vi "SP_Production_Count_MonthWise.vi"(8 "error in (no error)":errorcluster) -> (0 "error out":errorcluster)   [LabVIEW 2017]
uses:
  <vilib>/Math Plots/3D Math Plots/3D Pie/3D Pie XCtrl/3D Pie.xctl
  <vilib>/addons/database/Connection.llb/DB Tools Open Connec (Path).vi
  <vilib>/addons/database/Connection.llb/Conn Execute.vi
  <vilib>/addons/database/Recordset.llb/Rec Fetch Recordset Data (R).vi
  <vilib>/addons/database/Recordset.llb/Rec Destroy - Connection.vi
  <vilib>/Math Plots/3D Math Plots/3D Pie/3D Pie Datatype/Public/Plot Helper (Vector).vi
  <vilib>/addons/database/NI_Database_API.lvlib
  <vilib>/Math Plots/3D Math Plots/3D Pie/3D Pie Datatype/3D Pie Datatype.lvclass
panel:
  out "Station size":i32
  in  "Tab Control":enum32{"Data", "Graph"}(tab)
  out "Table":string[][](table)
  out "3D Pie":refnum<class "3D Plot Datatype.lvclass">[](xcontrol)
  out "All Days":string[](array[string])
  in  "Select Year":string(combo)
  in  "Select Month":string(combo)
  out "Station Count":i32
  out "All Shifts":bool
  in  "Cancel Button - Archive":bool
  in  "Download 2":bool
  in  "Get Rport 2":bool
  in  "Shift":string(combo)
  in  "Station":string(combo)
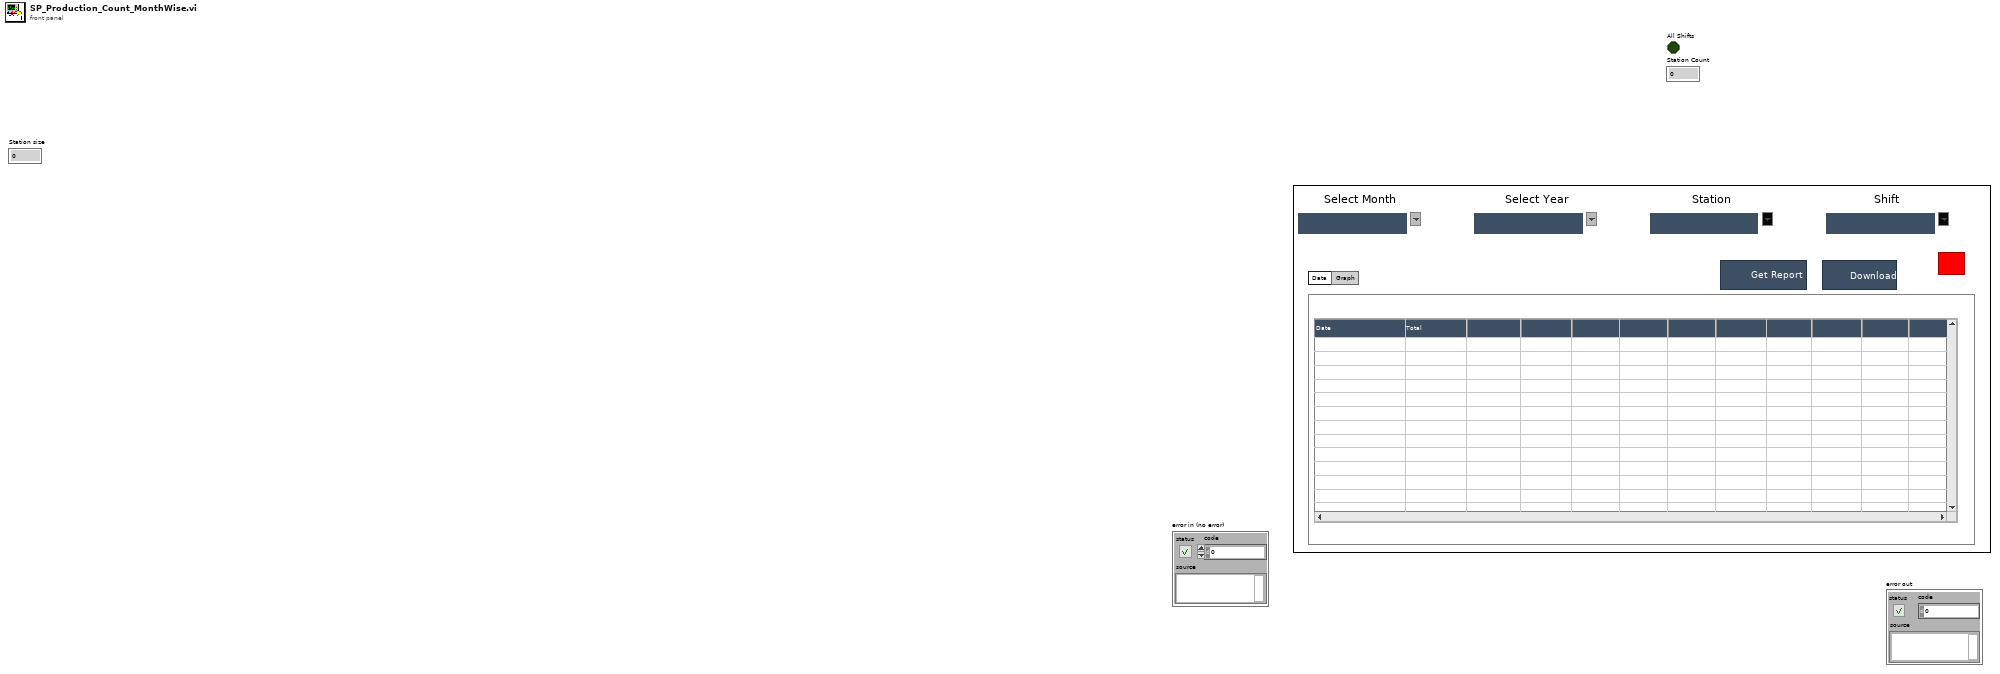
[diagram p1: front panel]
types:
  T1 = typedef "NI_Database_API.lvlib/Conn ObjectReference.ctl" = refnum<k1>
  T2 = typedef "NI_Database_API.lvlib/Rec ObjectReference.ctl" = refnum<k1>
  T3 = enum32{"invalid app kind", "Development System", "Run Time System", "Student Edition", "Embedded LabVIEW", "Evaluation", "Custom"}
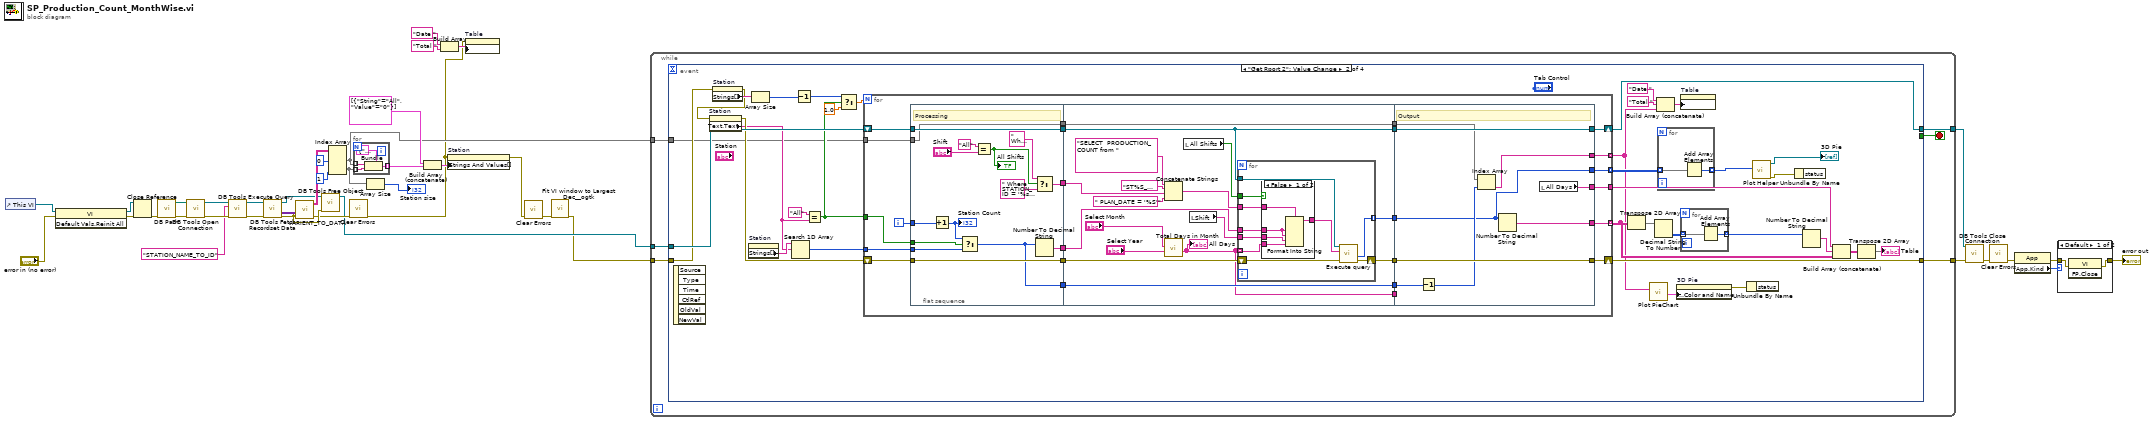
[diagram p0: block diagram]
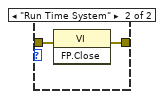
[diagram p2: hidden frame]
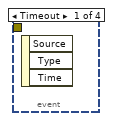
[diagram p3: hidden frame]
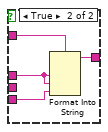
[diagram p4: hidden frame]
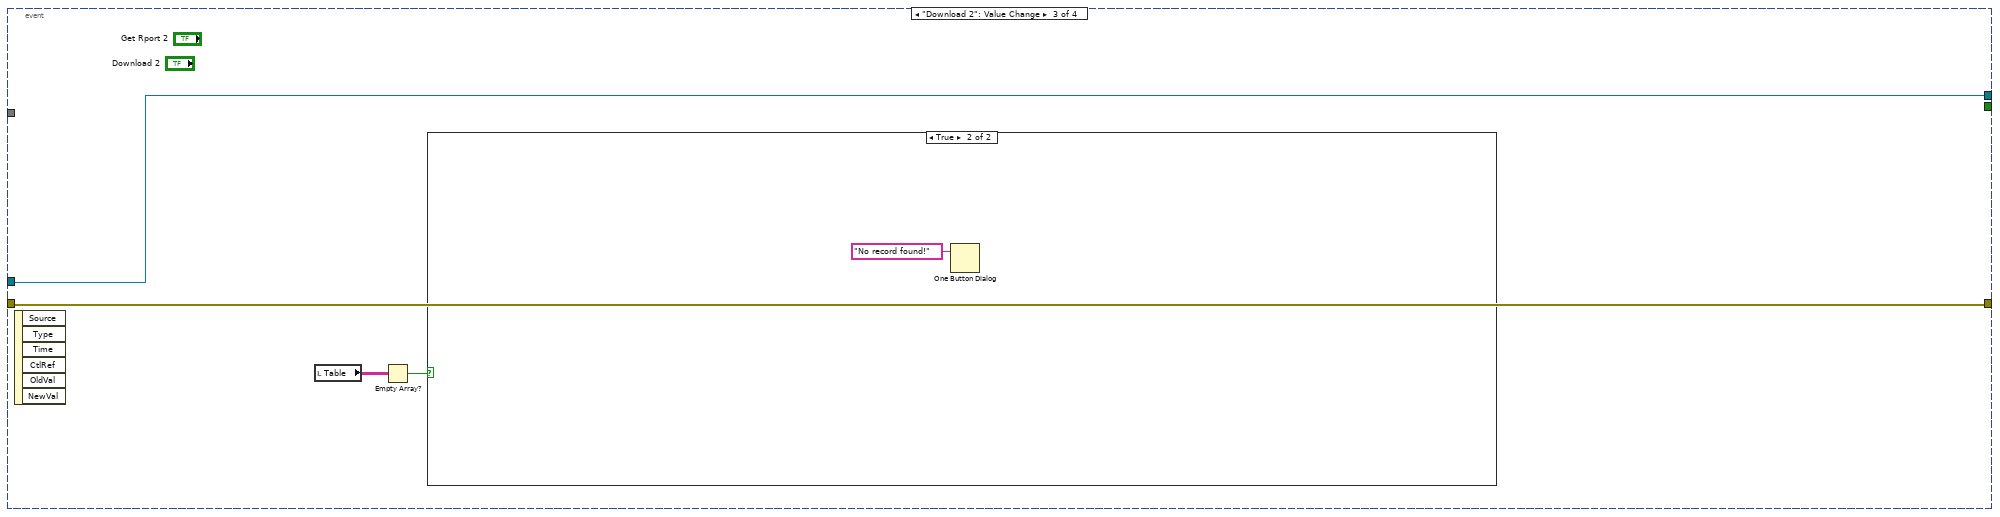
[diagram p5: hidden frame]
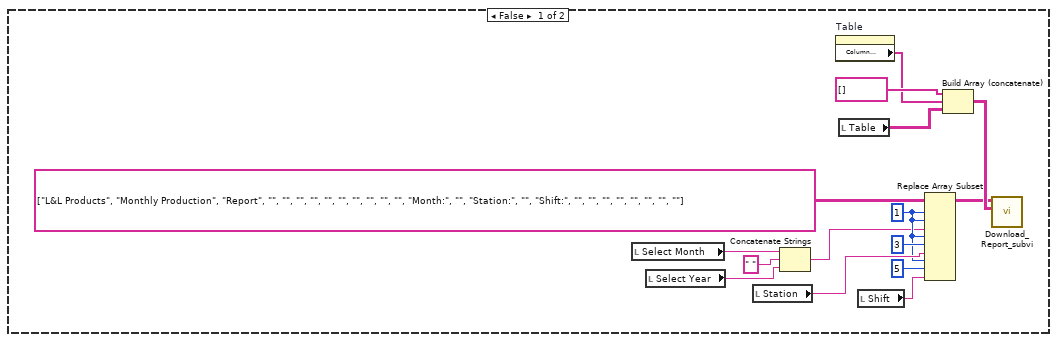
[diagram p6: hidden frame]
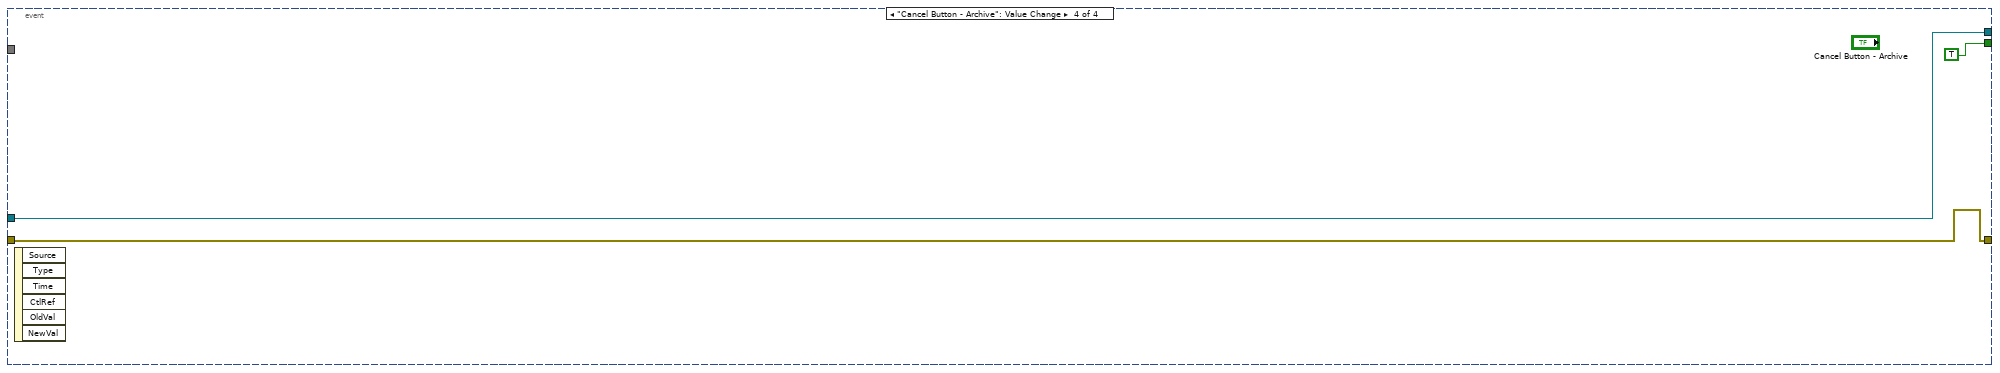
[diagram p7: hidden frame]
diagram:
  n1 = control-ref of="This VI"() -> (w33:refnum<vi>)
  n2 = invoke class="VI" method="Default Vals.Reinit All"(reference=w33, error in="error in (no error)") -> (reference out=w31:refnum<vi>, error out=w32:errorcluster)  [unwired: 1 in, 1 out]
  n3 = Close Reference(reference=w31, error in (no error)=w32) -> (error out=w30:errorcluster)
  n4 = call "DB Path.vi"("error in"=w30) -> ("error out"=w29:errorcluster, "DB Path"=w28:path)  [unwired: 9 in]
  n5 = call-poly <vilib>:"DB Tools Open Connection.vi"("error in (no error)"=w29, "connection information"=w28) -> ("error out"=w17:errorcluster, "connection reference"=w18:T1)  [unwired: 6 in]
  n6 = call-poly <vilib>:"DB Tools Execute Query.vi"("error in (no error)"=w17, "SQL query"="STATION_NAME_TO_ID", "connection reference"=w18) -> ("error out"=w26:errorcluster, "recordset reference"=w27:T2)  [unwired: 5 in]
  n7 = call-poly <vilib>:"DB Tools Fetch Recordset Data.vi"("error in (no error)"=w26, "recordset reference"=w27) -> ("error out"=w21:errorcluster, "recordset data"=w25:variant[][], "recordset reference out"=w19:T2)  [unwired: 3 in]
  n8 = call "VARIENT_TO_DATA.vi"("data"=w25, "error in (no error)"=w21) -> ("Table"=w22:string[][], "error out"=w20:errorcluster)  [unwired: 7 in]
  n9 = call-poly <vilib>:"DB Tools Free Object.vi"("error in (no error)"=w21, "recordset reference"=w19) -> ("connection reference"=w8:T1)  [unwired: 8 in, 1 out]
  n10 = Index Array(array=w22, index (col) #1=0 ("index (row)"), index (col) #2=1 ("index (col)")) -> (element #1=w5:string[], element #2=w12:string[])  [unwired: 2 in]
  n11 = call <vilib>:"Clear Errors.vi"("error in (no error)"=w20) -> ("error out"=w1:errorcluster)  [unwired: 5 in, 1 out]
  n12 = for {
    tunnel: w5 -> [w44] mode=indexing
    tunnel: w12 -> [w43] mode=indexing
    tunnel: [w41] -> w13 mode=indexing
    n13 = Bundle(cluster=cluster{"String":string, "Value":string} {"String"="", "Value"=""}, "String"=w44, "Value"=w43) -> (w41:cluster{"String":string, "Value":string})
  }
  n14 = Array Size(array=w12) -> (size(s)=→"Station size":i32)
  n15 = Build Array (concatenate)(cluster{"String":string, "Value":string}[] [{"String"="All", "Value"="0"}] ("array"), w13) -> (w15:cluster{"String":string, "Value":string}[])
  n16 = Build Array("Date ", "Total ") -> (w2:string[])
  n17 = property on="Station" class="CmbBox"(error in=w1, "Strings And Values[]"=w15) -> (error out=w9:errorcluster)  [unwired: 1 in, 1 out]
  n18 = property on="Table" class="Tbl (strict)"(error in=w1, "Column Headers[]"=w2) -> ()  [unwired: 1 in, 2 out]
  n19 = call <vilib>:"Clear Errors.vi"("error in (no error)"=w9) -> ("error out"=w10:errorcluster)  [unwired: 5 in, 1 out]
  n20 = call <userlib>:"Fit VI window to Largest Dec__ogtk.vi"("error in (no error)"=w10) -> ("error out"=w6:errorcluster)  [unwired: 5 in, 1 out]
  n21 = while {
    tunnel: w6 -> [w47]
    tunnel: w8 -> [w46]
    tunnel: [w49] -> w36
    tunnel: [w48] -> w35
    tunnel: w5 -> [w45]
    stop <- w50 stop-if-true
    n22 = event shown="[1] \"Get Rport 2\": Value Change" {
      selector: _ -> [_ _ _ _]
      dyn-events: _ -> [_ _ _ _]
      timeout: _ -> [_ _ _ _]
      tunnel: w46 -> [_ w85 w177 w195]
      tunnel: [_ _ _ TRUE] -> w50
      tunnel: [_ w83 w176 w194] -> w49
      tunnel: [_ w84 w177 w195] -> w48
      tunnel: w47 -> [_ w54 w176 w194]
      tunnel: w45 -> [_ w51 _ _]
      event Timeout {
        n23 = event-data() -> ()  [unwired: 1 in, 3 out]
      }
      event "Get Rport 2": Value Change {
        n24 = event-data() -> ()  [unwired: 1 in, 6 out]
        n25 = property on="Station" class="CmbBox"(error in=w54) -> (error out=w55:errorcluster, "Strings[]"=w79:string[])  [unwired: 1 in, 1 out]
        n26 = property on="Station" class="CmbBox"(error in=w55) -> (error out=w53:errorcluster, "Text.Text"=w52:string)  [unwired: 1 in, 1 out]
        n27 = property on="Station" class="CmbBox"() -> ("Strings[]"=w76:string[])  [unwired: 2 in, 2 out]
        n28 = Array Size(array=w79) -> (size(s)=w78:i32)
        n29 = Search 1D Array(1D array=w76, element=w52) -> (index of element=w74:i32)  [unwired: 1 in]
        n30 = Decrement(x=w78) -> (x-1=w77:i32)
        n31 = Equal?(x="All", y=w52) -> (x = y?=w75:bool)
        n32 = Select(t=w77, s=w75, f=1.0) -> (s? t:f=w81:dbl)
        n33 = for {
          N: w81 -> [_]
          shift-right: [w106] -> w84
          shift-left: w85 -> [w113]
          shift-right: [w107] -> w83
          shift-left: w53 -> [w112]
          tunnel: w75 -> [w111]
          tunnel: w74 -> [w110]
          tunnel: [w108] -> w56 mode=indexing
          tunnel: [w98] -> w67 mode=indexing
          tunnel: [w97] -> w70
          tunnel: [w94] -> w59 mode=indexing
          tunnel: w51 -> [w92]
          i -> [w109]
          n34 = flat-sequence {
            tunnel: [w125] -> w105
            tunnel: [w126] -> w103
            tunnel: [w128] -> w101
            tunnel: [w127] -> w100
            tunnel: w109 -> [w120]
            tunnel: w110 -> [w121]
            tunnel: w111 -> [w122]
            tunnel: w112 -> [w125]
            tunnel: w113 -> [w126]
            tunnel: [w115] -> w95
            tunnel: w92 -> [w114]
            tunnel: [w114] -> w90
            tunnel: w105 -> [w137]
            tunnel: [w136] -> w104
            tunnel: w103 -> [w138]
            tunnel: [w138] -> w102
            tunnel: w101 -> [w143]
            tunnel: w100 -> [w134]
            tunnel: [w135] -> w99
            tunnel: [w131] -> w96
            tunnel: w95 -> [w131]
            tunnel: [w130] -> w93
            tunnel: [w129] -> w91
            tunnel: w90 -> [w129]
            tunnel: [w167] -> w108
            tunnel: w104 -> [w170]
            tunnel: [w170] -> w107
            tunnel: [w173] -> w106
            tunnel: w102 -> [w173]
            tunnel: w99 -> [w166]
            tunnel: [w172] -> w98
            tunnel: [w171] -> w97
            tunnel: w96 -> [w169]
            tunnel: [w166] -> w94
            tunnel: w93 -> [_]
            tunnel: w91 -> [w165]
            frame #0 {
              # "Processing"
              n35 = Increment(x=w120) -> (x+1=w119:i32)
              "Station Count" <- w119
              n36 = Select(t=w119, s=w122, f=w121) -> (s? t:f=w115:i32)
              n37 = Equal?(x="All", y="Shift") -> (x = y?=w118:bool)
              "All Shifts" <- w118
              n38 = Select(t=" Where STATION_ID = '%s' and " ("format string"), s=w118, f=" Where STATION_ID = '%s' and SHIFT = '%s' and" ("format string")) -> (s? t:f=w128:string)
              n39 = Number To Decimal String(number=w115) -> (decimal integer string=w127:string)  [unwired: 1 in]
            }
            frame #1 {
              n40 = Concatenate Strings("SELECT  PRODUCTION_COUNT from " ("format string"), "ST%S_PRODUCTION_COUNT", w143, " PLAN_DATE = '%S'" ("string")) -> (w140:string)
              n41 = call "Total Days in Month.vi"("Year"="Select Year", "Month"="Select Month") -> ("All Days"=w130:string[])  [unwired: 8 in, 1 out]
              "All Days" <- w130
              n42 = local read "All Shifts"() -> (w141:bool)
              n43 = local read "Shift"() -> (w139:string)
              n44 = for {
                tunnel: w141 -> [w155]
                tunnel: w140 -> [w154]
                tunnel: w134 -> [w153]
                tunnel: w139 -> [w152]
                tunnel: w130 -> [w151] mode=indexing
                tunnel: w138 -> [w149]
                shift-right: [w147] -> w136
                shift-left: w137 -> [w148]
                tunnel: [w146] -> w135 mode=indexing
                n45 = case shown="False" w155 {
                  tunnel: w154 -> [w160 w164]
                  tunnel: w153 -> [w159 w163]
                  tunnel: w152 -> [w158 _]
                  tunnel: w151 -> [w157 w162]
                  tunnel: [w156 w161] -> w150
                  frame False {
                    n46 = Format Into String(format string=w160, w159, w159, w158, w157) -> (resulting string=w156:string)  [unwired: 2 in, 1 out]
                  }
                  frame True {
                    n47 = Format Into String(format string=w164, w163, w163, w162) -> (resulting string=w161:string)  [unwired: 2 in, 1 out]
                  }
                }
                n48 = call "Execute query.vi"("error in (no error)"=w148, "String"=w150, "connection reference"=w149) -> ("error out"=w147:errorcluster, "Production Count"=w146:i32)  [unwired: 3 in, 4 out]
              }
            }
            frame #2 {
              # "Output"
              n49 = Decrement(x=w169) -> (x-1=w168:i32)
              n50 = Index Array(array=w165, index=w168) -> (element=w167:string)
              n51 = Number To Decimal String(number=w166) -> (decimal integer string=w172:string[])  [unwired: 1 in]
              n52 = local read "All Days"() -> (w171:string[])
            }
          }
        }
        n53 = Transpose 2D Array(2D array=w67) -> (transposed array=w66:string[][])
        n54 = call "Plot PieChart.vi"("Label"=w56) -> ("Labelling"=w58:cluster{dbl, "String":string}[])  [unwired: 10 in]
        n55 = Decimal String To Number(string=w66) -> (number=w65:i32[][])  [unwired: 2 in, 1 out]
        n56 = Build Array (concatenate)("Date ", "Total ", w56) -> (w73:string[])
        n57 = for {
          tunnel: w59 -> [w87] mode=indexing
          tunnel: [w86] -> w61 mode=indexing
          n58 = Add Array Elements(numeric array=w87) -> (sum=w86:i32)
        }
        n59 = property on="3D Pie" class="3D Pie (strict)"("Plot Specific:Color and Name"=w58) -> (error out=w57:errorcluster)  [unwired: 2 in, 1 out]
        n60 = property on="Table" class="Tbl (strict)"("Column Headers[]"=w73) -> ()  [unwired: 2 in, 2 out]
        n61 = for {
          tunnel: w65 -> [w89] mode=indexing
          tunnel: [w88] -> w64 mode=indexing
          n62 = Add Array Elements(numeric array=w89) -> (sum=w88:i32)
        }
        n63 = Unbundle By Name(w57) -> ()  [unwired: 1 out]
        n64 = call-poly <vilib>:"Plot Helper.vi"("x vector"=w61) -> ("error out"=w62:errorcluster, "3D Plot lvclass Array out"=→"3D Pie":refnum<class "3D Plot Datatype.lvclass">[])  [unwired: 2 in, 7 out]
        n65 = Unbundle By Name(w62) -> ()  [unwired: 1 out]
        n66 = Number To Decimal String(number=w64) -> (decimal integer string=w63:string[])  [unwired: 1 in]
        n67 = Build Array (concatenate)(w70, w63, w67) -> (w72:string[][])
        n68 = Transpose 2D Array(2D array=w72) -> (transposed array=→"Table":string[][])
      }
      event "Download 2": Value Change {
        n69 = event-data() -> ()  [unwired: 1 in, 6 out]
        n70 = local read "Table"() -> (w175:string[][])
        n71 = Empty Array?(array=w175) -> (empty?=w174:bool)
        n72 = case shown="True" w174 {
          frame False {
            w189 = 1 ("index (row)")
            n73 = local read "Select Month"() -> (w186:string)
            n74 = local read "Select Year"() -> (w185:string)
            n75 = local read "Station"() -> (w190:string)
            n76 = Concatenate Strings(w186, " " ("string"), w185) -> (w184:string)
            n77 = property on="Table" class="Tbl (strict)"() -> ("Column Headers[]"=w179:string[])  [unwired: 2 in, 2 out]
            n78 = local read "Table"() -> (w181:string[][])
            n79 = local read "Shift"() -> (w187:string)
            n80 = Replace Array Subset(array=string[][] [["L&L Products", "Monthly Production", "Report", "", "", "", "", "", "", "", "", "", ""], ["Month:", "", "Station:", "", "Shift:", "", "", "", "", "", "", "", ""]] ("Column Header Strings[]"), new element #1=w184, index (row) #1=w189, index (col) #1=w189, new element #2=w190, index (row) #2=w189, index (col) #2=3 ("disabled index (col)"), new element #3=w187, index (row) #3=w189, index (col) #3=5 ("disabled index (col)")) -> (w178:string[][])
            n81 = Build Array (concatenate)(string[] [] ("element"), w179, w181) -> (w180:string[][])
            n82 = call "Download_Report_subvi.vi"("Value"=w180, "Column Header Strings[]"=w178) -> ()  [unwired: 9 in, 1 out]
          }
          frame True {
            n83 = One Button Dialog(message="No record found!") -> ()  [unwired: 1 in, 1 out]
          }
        }
      }
      event "Cancel Button - Archive": Value Change {
        n84 = event-data() -> ()  [unwired: 1 in, 6 out]
      }
    }
  }
  n85 = call <vilib>:"DB Tools Close Connection.vi"("error in (no error)"=w36, "connection reference"=w35) -> ("error out"=w38:errorcluster)  [unwired: 5 in]
  n86 = call <vilib>:"Clear Errors.vi"("error in (no error)"=w38) -> ("error out"=w37:errorcluster)  [unwired: 5 in, 1 out]
  n87 = property class="App"(error in=w37) -> (error out=w39:errorcluster, "App.Kind"=w40:T3)  [unwired: 1 in, 1 out]
  n88 = case shown="Default" w40 {
    tunnel: w39 -> [w198 w200]
    tunnel: [w197 w199] -> w34
    frame Default {
      n89 = invoke class="VI" method="FP.Close"(error in=w198) -> (error out=w197:errorcluster)  [unwired: 2 in, 2 out]
    }
    frame "Run Time System" {
      n90 = invoke class="VI" method="FP.Close"(error in=w200) -> (error out=w199:errorcluster)  [unwired: 2 in, 2 out]
    }
  }
  "error out" <- w34
